vi "ReadWindVane.vi"(8 "Error in":errorcluster) -> (0 "error out":errorcluster, 3 "Measured wind angle":dbl)   [LabVIEW 2013]
uses:
  <vilib>/measure/mascope.llb/Pulse Measurements 1 chan.vi
  <vilib>/measure/NI_MAPro.lvlib
panel:
  out "pulse duration":dbl format="%.2g"
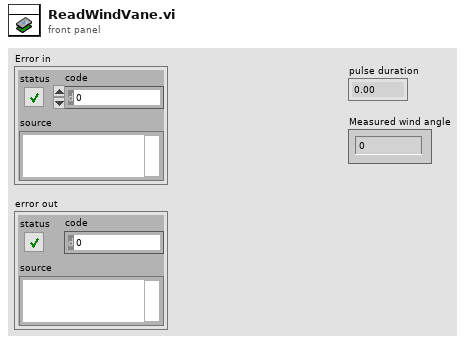
[diagram p1: front panel]
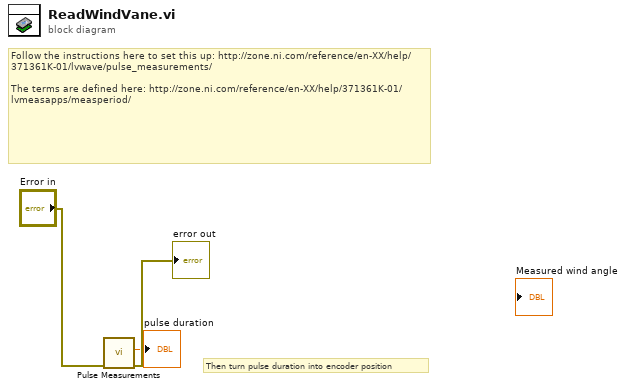
[diagram p0: block diagram]
diagram:
  # "Then turn pulse duration into encoder position"
  # "Follow the instructions here to set this up: http://zone.ni.com/reference/en-XX/help/371361K-01/lvwave/pulse_measurements/\n\nThe terms are defined here: http://zone.ni.com/reference/en-XX/help/371361K-01/lvmeasapps/measperiod/"
  n1 = call-poly <vilib>:"Pulse Measurements.vi"("error in (no error)"="Error in") -> ("error out"=→"error out":errorcluster, "pulse duration"=→"pulse duration":dbl)  [unwired: 6 in, 3 out]
